vi "Stop Control Panel.vi"(8 "error in (no error)":errorcluster, 9 "timeout in ms (-1)":i32=-1, 10 "Blocking (T)":bool=TRUE, 11 "controller in":refnum<class "Generic Plugin.lvclass">) -> (0 "error out":errorcluster, 3 "controller out":refnum<class "Generic Plugin.lvclass">)   [LabVIEW 2020, in "RxnRover.lvlib" / "Generic Plugin.lvclass"]
doc: "Sends the \"Exit\" command to the associated control panel. By default, this VI blocks until the \"Process Exit\" command is received from the control panel."
uses:
  Generic Plugin.lvclass
  Generic Plugin.lvclass/Generic Plugin.ctl
  <userlib>/RxnRover/DynamicReentrant/Dynamic Reentrant.lvlib
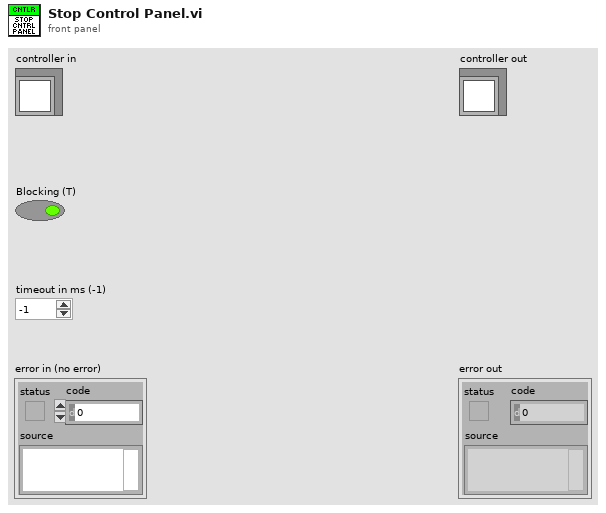
[diagram p1: front panel]
types:
  T1 = typedef "Dynamic Reentrant.lvlib/Message.ctl" = cluster{"Source":string, "Destination":string, "Time Stamp":timestamp, "Command":string, "Data":variant}
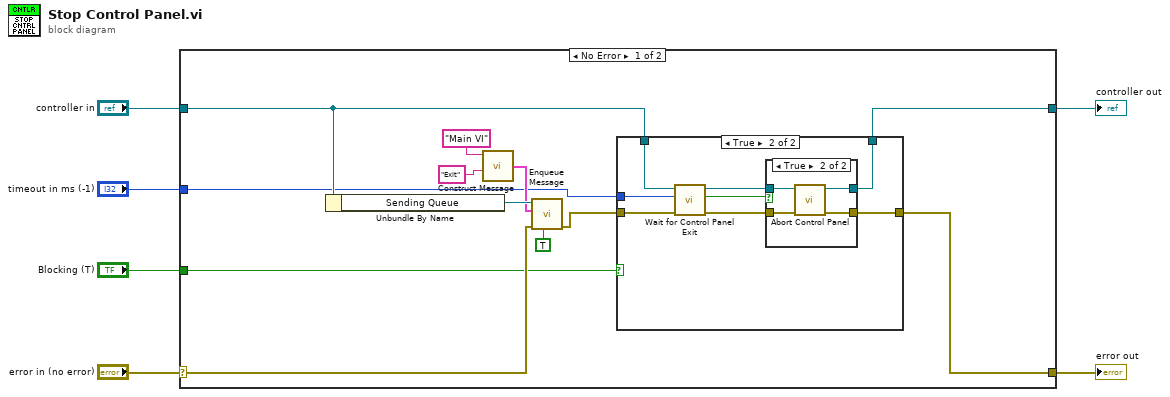
[diagram p0: block diagram]
diagram:
  n1 = case shown="No Error" "error in (no error)" {
    selector: "error in (no error)" -> [w14 w36]
    tunnel: [w10 w36] -> w5
    tunnel: [w12 w35] -> w3
    tunnel: "controller in" -> [w13 w35]
    tunnel: "Blocking (T)" -> [w11 _]
    tunnel: "timeout in ms (-1)" -> [w7 _]
    frame No Error {
      n2 = Unbundle By Name(w13) -> ("Sending Queue"=w18:refnum<queue>)
      n3 = call <userlib>:"Construct Message.vi"("Command"="Exit", "Source"="Main VI") -> ("Message Cluster"=w8:T1)  [unwired: 4 in]
      n4 = call <userlib>:"Enqueue Message.vi"("Priority Message? (F)"=TRUE, "error in (no error)"=w14, "Message"=w8, "Listening Queue"=w18) -> ("error out"=w15:errorcluster)  [unwired: 6 in, 1 out]
      n5 = case shown="True" w11 {
        tunnel: w15 -> [w19 w28]
        tunnel: w13 -> [w20 w27]
        tunnel: [w20 w21] -> w12
        tunnel: [w19 w24] -> w10
        tunnel: w7 -> [_ w25]
        frame False {
        }
        frame True {
          n6 = call "Wait for Control Panel Exit.vi"("error in (no error)"=w28, "timeout in ms (-1)"=w25, "Generic Controller in"=w27) -> ("error out"=w26:errorcluster, "Timeout?"=w23:bool, "Generic Controller out"=w22:refnum<class "Generic Plugin.lvclass">)  [unwired: 6 in]
          n7 = case shown="True" w23 {
            tunnel: w26 -> [w29 w34]
            tunnel: [w29 w33] -> w24
            tunnel: w22 -> [w30 w32]
            tunnel: [w30 w31] -> w21
            frame False {
            }
            frame True {
              n8 = call "Abort Control Panel.vi"("error in (no error)"=w34, "Generic Controller in"=w32) -> ("error out"=w33:errorcluster, "Generic Controller out"=w31:refnum<class "Generic Plugin.lvclass">)  [unwired: 8 in]
            }
          }
        }
      }
    }
    frame Error {
    }
  }
  "error out" <- w5
  "controller out" <- w3
